vi "FipsAdjacent.vi"() -> (11 "Fips":i32[](array[numeric]))   [LabVIEW 2017] (continued)
 County, KY\"\t21075\t\"Hickman County, KY\"\t21105\n\"Fulton County, KY\"\t21075\t\"Mississippi County, MO\"\t29133\n\"Fulton County, KY\"\t21075\t\"New Madrid County, MO\"\t29143\n\"Fulton County, KY\"\t21075\t\"Lake County, TN\"\t47095\n\"Fulton County, KY\"\t21075\t\"Obion County, TN\"\t47131\n\"Gallatin County, KY\"\t21077\t\"Switzerland County, IN\"\t18155\n\"Gallatin County, KY\"\t21077\t\"Boone County, KY\"\t21015\n\"Gallatin County, KY\"\t21077\t\"Carroll County, KY\"\t21041\n\"Gallatin County, KY\"\t21077\t\"Gallatin County, KY\"\t21077\n\"Gallatin County, KY\"\t21077\t\"Grant County, KY\"\t21081\n\"Gallatin County, KY\"\t21077\t\"Owen County, KY\"\t21187\n\"Garrard County, KY\"\t21079\t\"Boyle County, KY\"\t21021\n\"Garrard County, KY\"\t21079\t\"Garrard County, KY\"\t21079\n\"Garrard County, KY\"\t21079\t\"Jessamine County, KY\"\t21113\n\"Garrard County, KY\"\t21079\t\"Lincoln County, KY\"\t21137\n\"Garrard County, KY\"\t21079\t\"Madison County, KY\"\t21151\n\"Garrard County, KY\"\t21079\t\"Mercer County, KY\"\t21167\n\"Garrard County, KY\"\t21079\t\"Rockcastle County, KY\"\t21203\n\"Grant County, KY\"\t21081\t\"Boone County, KY\"\t21015\n\"Grant County, KY\"\t21081\t\"Gallatin County, KY\"\t21077\n\"Grant County, KY\"\t21081\t\"Grant County, KY\"\t21081\n\"Grant County, KY\"\t21081\t\"Harrison County, KY\"\t21097\n\"Grant County, KY\"\t21081\t\"Kenton County, KY\"\t21117\n\"Grant County, KY\"\t21081\t\"Owen County, KY\"\t21187\n\"Grant County, KY\"\t21081\t\"Pendleton County, KY\"\t21191\n\"Grant County, KY\"\t21081\t\"Scott County, KY\"\t21209\n\"Graves County, KY\"\t21083\t\"Calloway County, KY\"\t21035\n\"Graves County, KY\"\t21083\t\"Carlisle County, KY\"\t21039\n\"Graves County, KY\"\t21083\t\"Graves County, KY\"\t21083\n\"Graves County, KY\"\t21083\t\"Hickman County, KY\"\t21105\n\"Graves County, KY\"\t21083\t\"McCracken County, KY\"\t21145\n\"Graves County, KY\"\t21083\t\"Marshall County, KY\"\t21157\n\"Graves County, KY\"\t21083\t\"Henry County, TN\"\t47079\n\"Graves County, KY\"\t21083\t\"Weakley County, TN\"\t47183\n\"Grayson County, KY\"\t21085\t\"Breckinridge County, KY\"\t21027\n\"Grayson County, KY\"\t21085\t\"Butler County, KY\"\t21031\n\"Grayson County, KY\"\t21085\t\"Edmonson County, KY\"\t21061\n\"Grayson County, KY\"\t21085\t\"Grayson County, KY\"\t21085\n\"Grayson County, KY\"\t21085\t\"Hardin County, KY\"\t21093\n\"Grayson County, KY\"\t21085\t\"Hart County, KY\"\t21099\n\"Grayson County, KY\"\t21085\t\"Ohio County, KY\"\t21183\n\"Green County, KY\"\t21087\t\"Adair County, KY\"\t21001\n\"Green County, KY\"\t21087\t\"Green County, KY\"\t21087\n\"Green County, KY\"\t21087\t\"Hart County, KY\"\t21099\n\"Green County, KY\"\t21087\t\"Larue County, KY\"\t21123\n\"Green County, KY\"\t21087\t\"Metcalfe County, KY\"\t21169\n\"Green County, KY\"\t21087\t\"Taylor County, KY\"\t21217\n\"Greenup County, KY\"\t21089\t\"Boyd County, KY\"\t21019\n\"Greenup County, KY\"\t21089\t\"Carter County, KY\"\t21043\n\"Greenup County, KY\"\t21089\t\"Greenup County, KY\"\t21089\n\"Greenup County, KY\"\t21089\t\"Lewis County, KY\"\t21135\n\"Greenup County, KY\"\t21089\t\"Lawrence County, OH\"\t39087\n\"Greenup County, KY\"\t21089\t\"Scioto County, OH\"\t39145\n\"Hancock County, KY\"\t21091\t\"Perry County, IN\"\t18123\n\"Hancock County, KY\"\t21091\t\"Spencer County, IN\"\t18147\n\"Hancock County, KY\"\t21091\t\"Breckinridge County, KY\"\t21027\n\"Hancock County, KY\"\t21091\t\"Daviess County, KY\"\t21059\n\"Hancock County, KY\"\t21091\t\"Hancock County, KY\"\t21091\n\"Hancock County, KY\"\t21091\t\"Ohio County, KY\"\t21183\n\"Hardin County, KY\"\t21093\t\"Harrison County, IN\"\t18061\n\"Hardin County, KY\"\t21093\t\"Breckinridge County, KY\"\t21027\n\"Hardin County, KY\"\t21093\t\"Bullitt County, KY\"\t21029\n\"Hardin County, KY\"\t21093\t\"Grayson County, KY\"\t21085\n\"Hardin County, KY\"\t21093\t\"Hardin County, KY\"\t21093\n\"Hardin County, KY\"\t21093\t\"Hart County, KY\"\t21099\n\"Hardin County, KY\"\t21093\t\"Jefferson County, KY\"\t21111\n\"Hardin County, KY\"\t21093\t\"Larue County, KY\"\t21123\n\"Hardin County, KY\"\t21093\t\"Meade County, KY\"\t21163\n\"Hardin County, KY\"\t21093\t\"Nelson County, KY\"\t21179\n\"Harlan County, KY\"\t21095\t\"Bell County, KY\"\t21013\n\"Harlan County, KY\"\t21095\t\"Harlan County, KY\"\t21095\n\"Harlan County, KY\"\t21095\t\"Leslie County, KY\"\t21131\n\"Harlan County, KY\"\t21095\t\"Letcher County, KY\"\t21133\n\"Harlan County, KY\"\t21095\t\"Perry County, KY\"\t21193\n\"Harlan County, KY\"\t21095\t\"Lee County, VA\"\t51105\n\"Harlan County, KY\"\t21095\t\"Wise County, VA\"\t51195\n\"Harrison County, KY\"\t21097\t\"Bourbon County, KY\"\t21017\n\"Harrison County, KY\"\t21097\t\"Bracken County, KY\"\t21023\n\"Harrison County, KY\"\t21097\t\"Grant County, KY\"\t21081\n\"Harrison County, KY\"\t21097\t\"Harrison County, KY\"\t21097\n\"Harrison County, KY\"\t21097\t\"Nicholas County, KY\"\t21181\n\"Harrison County, KY\"\t21097\t\"Pendleton County, KY\"\t21191\n\"Harrison County, KY\"\t21097\t\"Robertson County, KY\"\t21201\n\"Harrison County, KY\"\t21097\t\"Scott County, KY\"\t21209\n\"Hart County, KY\"\t21099\t\"Barren County, KY\"\t21009\n\"Hart County, KY\"\t21099\t\"Edmonson County, KY\"\t21061\n\"Hart County, KY\"\t21099\t\"Grayson County, KY\"\t21085\n\"Hart County, KY\"\t21099\t\"Green County, KY\"\t21087\n\"Hart County, KY\"\t21099\t\"Hardin County, KY\"\t21093\n\"Hart County, KY\"\t21099\t\"Hart County, KY\"\t21099\n\"Hart County, KY\"\t21099\t\"Larue County, KY\"\t21123\n\"Hart County, KY\"\t21099\t\"Metcalfe County, KY\"\t21169\n\"Henderson County, KY\"\t21101\t\"Posey County, IN\"\t18129\n\"Henderson County, KY\"\t21101\t\"Vanderburgh County, IN\"\t18163\n\"Henderson County, KY\"\t21101\t\"Warrick County, IN\"\t18173\n\"Henderson County, KY\"\t21101\t\"Daviess County, KY\"\t21059\n\"Henderson County, KY\"\t21101\t\"Henderson County, KY\"\t21101\n\"Henderson County, KY\"\t21101\t\"McLean County, KY\"\t21149\n\"Henderson County, KY\"\t21101\t\"Union County, KY\"\t21225\n\"Henderson County, KY\"\t21101\t\"Webster County, KY\"\t21233\n\"Henry County, KY\"\t21103\t\"Carroll County, KY\"\t21041\n\"Henry County, KY\"\t21103\t\"Franklin County, KY\"\t21073\n\"Henry County, KY\"\t21103\t\"Henry County, KY\"\t21103\n\"Henry County, KY\"\t21103\t\"Oldham County, KY\"\t21185\n\"Henry County, KY\"\t21103\t\"Owen County, KY\"\t21187\n\"Henry County, KY\"\t21103\t\"Shelby County, KY\"\t21211\n\"Henry County, KY\"\t21103\t\"Trimble County, KY\"\t21223\n\"Hickman County, KY\"\t21105\t\"Carlisle County, KY\"\t21039\n\"Hickman County, KY\"\t21105\t\"Fulton County, KY\"\t21075\n\"Hickman County, KY\"\t21105\t\"Graves County, KY\"\t21083\n\"Hickman County, KY\"\t21105\t\"Hickman County, KY\"\t21105\n\"Hickman County, KY\"\t21105\t\"Mississippi County, MO\"\t29133\n\"Hickman County, KY\"\t21105\t\"Obion County, TN\"\t47131\n\"Hickman County, KY\"\t21105\t\"Weakley County, TN\"\t47183\n\"Hopkins County, KY\"\t21107\t\"Caldwell County, KY\"\t21033\n\"Hopkins County, KY\"\t21107\t\"Christian County, KY\"\t21047\n\"Hopkins County, KY\"\t21107\t\"Hopkins County, KY\"\t21107\n\"Hopkins County, KY\"\t21107\t\"McLean County, KY\"\t21149\n\"Hopkins County, KY\"\t21107\t\"Muhlenberg County, KY\"\t21177\n\"Hopkins County, KY\"\t21107\t\"Webster County, KY\"\t21233\n\"Jackson County, KY\"\t21109\t\"Clay County, KY\"\t21051\n\"Jackson County, KY\"\t21109\t\"Estill County, KY\"\t21065\n\"Jackson County, KY\"\t21109\t\"Jackson County, KY\"\t21109\n\"Jackson County, KY\"\t21109\t\"Laurel County, KY\"\t21125\n\"Jackson County, KY\"\t21109\t\"Lee County, KY\"\t21129\n\"Jackson County, KY\"\t21109\t\"Madison County, KY\"\t21151\n\"Jackson County, KY\"\t21109\t\"Owsley County, KY\"\t21189\n\"Jackson County, KY\"\t21109\t\"Rockcastle County, KY\"\t21203\n\"Jefferson County, KY\"\t21111\t\"Clark County, IN\"\t18019\n\"Jefferson County, KY\"\t21111\t\"Floyd County, IN\"\t18043\n\"Jefferson County, KY\"\t21111\t\"Harrison County, IN\"\t18061\n\"Jefferson County, KY\"\t21111\t\"Bullitt County, KY\"\t21029\n\"Jefferson County, KY\"\t21111\t\"Hardin County, KY\"\t21093\n\"Jefferson County, KY\"\t21111\t\"Jefferson County, KY\"\t21111\n\"Jefferson County, KY\"\t21111\t\"Oldham County, KY\"\t21185\n\"Jefferson County, KY\"\t21111\t\"Shelby County, KY\"\t21211\n\"Jefferson County, KY\"\t21111\t\"Spencer County, KY\"\t21215\n\"Jessamine County, KY\"\t21113\t\"Fayette County, KY\"\t21067\n\"Jessamine County, KY\"\t21113\t\"Garrard County, KY\"\t21079\n\"Jessamine County, KY\"\t21113\t\"Jessamine County, KY\"\t21113\n\"Jessamine County, KY\"\t21113\t\"Madison County, KY\"\t21151\n\"Jessamine County, KY\"\t21113\t\"Mercer County, KY\"\t21167\n\"Jessamine County, KY\"\t21113\t\"Woodford County, KY\"\t21239\n\"Johnson County, KY\"\t21115\t\"Floyd County, KY\"\t21071\n\"Johnson County, KY\"\t21115\t\"Johnson County, KY\"\t21115\n\"Johnson County, KY\"\t21115\t\"Lawrence County, KY\"\t21127\n\"Johnson County, KY\"\t21115\t\"Magoffin County, KY\"\t21153\n\"Johnson County, KY\"\t21115\t\"Martin County, KY\"\t21159\n\"Johnson County, KY\"\t21115\t\"Morgan County, KY\"\t21175\n\"Kenton County, KY\"\t21117\t\"Boone County, KY\"\t21015\n\"Kenton County, KY\"\t21117\t\"Campbell County, KY\"\t21037\n\"Kenton County, KY\"\t21117\t\"Grant County, KY\"\t21081\n\"Kenton County, KY\"\t21117\t\"Kenton County, KY\"\t21117\n\"Kenton County, KY\"\t21117\t\"Pendleton County, KY\"\t21191\n\"Kenton County, KY\"\t21117\t\"Hamilton County, OH\"\t39061\n\"Knott County, KY\"\t21119\t\"Breathitt County, KY\"\t21025\n\"Knott County, KY\"\t21119\t\"Floyd County, KY\"\t21071\n\"Knott County, KY\"\t21119\t\"Knott County, KY\"\t21119\n\"Knott County, KY\"\t21119\t\"Letcher County, KY\"\t21133\n\"Knott County, KY\"\t21119\t\"Magoffin County, KY\"\t21153\n\"Knott County, KY\"\t21119\t\"Perry County, KY\"\t21193\n\"Knott County, KY\"\t21119\t\"Pike County, KY\"\t21195\n\"Knox County, KY\"\t21121\t\"Bell County, KY\"\t21013\n\"Knox County, KY\"\t21121\t\"Clay County, KY\"\t21051\n\"Knox County, KY\"\t21121\t\"Knox County, KY\"\t21121\n\"Knox County, KY\"\t21121\t\"Laurel County, KY\"\t21125\n\"Knox County, KY\"\t21121\t\"Whitley County, KY\"\t21235\n\"Larue County, KY\"\t21123\t\"Green County, KY\"\t21087\n\"Larue County, KY\"\t21123\t\"Hardin County, KY\"\t21093\n\"Larue County, KY\"\t21123\t\"Hart County, KY\"\t21099\n\"Larue County, KY\"\t21123\t\"Larue County, KY\"\t21123\n\"Larue County, KY\"\t21123\t\"Marion County, KY\"\t21155\n\"Larue County, KY\"\t21123\t\"Nelson County, KY\"\t21179\n\"Larue County, KY\"\t21123\t\"Taylor County, KY\"\t21217\n\"Laurel County, KY\"\t21125\t\"Clay County, KY\"\t21051\n\"Laurel County, KY\"\t21125\t\"Jackson County, KY\"\t21109\n\"Laurel County, KY\"\t21125\t\"Knox County, KY\"\t21121\n\"Laurel County, KY\"\t21125\t\"Laurel County, KY\"\t21125\n\"Laurel County, KY\"\t21125\t\"McCreary County, KY\"\t21147\n\"Laurel County, KY\"\t21125\t\"Pulaski County, KY\"\t21199\n\"Laurel County, KY\"\t21125\t\"Rockcastle County, KY\"\t21203\n\"Laurel County, KY\"\t21125\t\"Whitley County, KY\"\t21235\n\"Lawrence County, KY\"\t21127\t\"Boyd County, KY\"\t21019\n\"Lawrence County, KY\"\t21127\t\"Carter County, KY\"\t21043\n\"Lawrence County, KY\"\t21127\t\"Elliott County, KY\"\t21063\n\"Lawrence County, KY\"\t21127\t\"Johnson County, KY\"\t21115\n\"Lawrence County, KY\"\t21127\t\"Lawrence County, KY\"\t21127\n\"Lawrence County, KY\"\t21127\t\"Martin County, KY\"\t21159\n\"Lawrence County, KY\"\t21127\t\"Morgan County, KY\"\t21175\n\"Lawrence County, KY\"\t21127\t\"Wayne County, WV\"\t54099\n\"Lee County, KY\"\t21129\t\"Breathitt County, KY\"\t21025\n\"Lee County, KY\"\t21129\t\"Estill County, KY\"\t21065\n\"Lee County, KY\"\t21129\t\"Jackson County, KY\"\t21109\n\"Lee County, KY\"\t21129\t\"Lee County, KY\"\t21129\n\"Lee County, KY\"\t21129\t\"Owsley County, KY\"\t21189\n\"Lee County, KY\"\t21129\t\"Powell County, KY\"\t21197\n\"Lee County, KY\"\t21129\t\"Wolfe County, KY\"\t21237\n\"Leslie County, KY\"\t21131\t\"Bell County, KY\"\t21013\n\"Leslie County, KY\"\t21131\t\"Clay County, KY\"\t21051\n\"Leslie County, KY\"\t21131\t\"Harlan County, KY\"\t21095\n\"Leslie County, KY\"\t21131\t\"Leslie County, KY\"\t21131\n\"Leslie County, KY\"\t21131\t\"Perry County, KY\"\t21193\n\"Letcher County, KY\"\t21133\t\"Harlan County, KY\"\t21095\n\"Letcher County, KY\"\t21133\t\"Knott County, KY\"\t21119\n\"Letcher County, KY\"\t21133\t\"Letcher County, KY\"\t21133\n\"Letcher County, KY\"\t21133\t\"Perry County, KY\"\t21193\n\"Letcher County, KY\"\t21133\t\"Pike County, KY\"\t21195\n\"Letcher County, KY\"\t21133\t\"Wise County, VA\"\t51195\n\"Lewis County, KY\"\t21135\t\"Carter County, KY\"\t21043\n\"Lewis County, KY\"\t21135\t\"Fleming County, KY\"\t21069\n\"Lewis County, KY\"\t21135\t\"Greenup County, KY\"\t21089\n\"Lewis County, KY\"\t21135\t\"Lewis County, KY\"\t21135\n\"Lewis County, KY\"\t21135\t\"Mason County, KY\"\t21161\n\"Lewis County, KY\"\t21135\t\"Rowan County, KY\"\t21205\n\"Lewis County, KY\"\t21135\t\"Adams County, OH\"\t39001\n\"Lewis County, KY\"\t21135\t\"Scioto County, OH\"\t39145\n\"Lincoln County, KY\"\t21137\t\"Boyle County, KY\"\t21021\n\"Lincoln County, KY\"\t21137\t\"Casey County, KY\"\t21045\n\"Lincoln County, KY\"\t21137\t\"Garrard County, KY\"\t21079\n\"Lincoln County, KY\"\t21137\t\"Lincoln County, KY\"\t21137\n\"Lincoln County, KY\"\t21137\t\"Pulaski County, KY\"\t21199\n\"Lincoln County, KY\"\t21137\t\"Rockcastle County, KY\"\t21203\n\"Livingston County, KY\"\t21139\t\"Hardin County, IL\"\t17069\n\"Livingston County, KY\"\t21139\t\"Massac County, IL\"\t17127\n\"Livingston County, KY\"\t21139\t\"Pope County, IL\"\t17151\n\"Livingston County, KY\"\t21139\t\"Crittenden County, KY\"\t21055\n\"Livingston County, KY\"\t21139\t\"Livingston County, KY\"\t21139\n\"Livingston County, KY\"\t21139\t\"Lyon County, KY\"\t21143\n\"Livingston County, KY\"\t21139\t\"McCracken County, KY\"\t21145\n\"Livingston County, KY\"\t21139\t\"Marshall County, KY\"\t21157\n\"Logan County, KY\"\t21141\t\"Butler County, KY\"\t21031\n\"Logan County, KY\"\t21141\t\"Logan County, KY\"\t21141\n\"Logan County, KY\"\t21141\t\"Muhlenberg County, KY\"\t21177\n\"Logan County, KY\"\t21141\t\"Simpson County, KY\"\t21213\n\"Logan County, KY\"\t21141\t\"Todd County, KY\"\t21219\n\"Logan County, KY\"\t21141\t\"Warren County, KY\"\t21227\n\"Logan County, KY\"\t21141\t\"Robertson County, TN\"\t47147\n\"Lyon County, KY\"\t21143\t\"Caldwell County, KY\"\t21033\n\"Lyon County, KY\"\t21143\t\"Crittenden County, KY\"\t21055\n\"Lyon County, KY\"\t21143\t\"Livingston County, KY\"\t21139\n\"Lyon County, KY\"\t21143\t\"Lyon County, KY\"\t21143\n\"Lyon County, KY\"\t21143\t\"Marshall County, KY\"\t21157\n\"Lyon County, KY\"\t21143\t\"Trigg County, KY\"\t21221\n\"McCracken County, KY\"\t21145\t\"Massac County, IL\"\t17127\n\"McCracken County, KY\"\t21145\t\"Pulaski County, IL\"\t17153\n\"McCracken County, KY\"\t21145\t\"Ballard County, KY\"\t21007\n\"McCracken County, KY\"\t21145\t\"Carlisle County, KY\"\t21039\n\"McCracken County, KY\"\t21145\t\"Graves County, KY\"\t21083\n\"McCracken County, KY\"\t21145\t\"Livingston County, KY\"\t21139\n\"McCracken County, KY\"\t21145\t\"McCracken County, KY\"\t21145\n\"McCracken County, KY\"\t21145\t\"Marshall County, KY\"\t21157\n\"McCreary County, KY\"\t21147\t\"Laurel County, KY\"\t21125\n\"McCreary County, KY\"\t21147\t\"McCreary County, KY\"\t21147\n\"McCreary County, KY\"\t21147\t\"Pulaski County, KY\"\t21199\n\"McCreary County, KY\"\t21147\t\"Wayne County, KY\"\t21231\n\"McCreary County, KY\"\t21147\t\"Whitley County, KY\"\t21235\n\"McCreary County, KY\"\t21147\t\"Campbell County, TN\"\t47013\n\"McCreary County, KY\"\t21147\t\"Scott County, TN\"\t47151\n\"McLean County, KY\"\t21149\t\"Daviess County, KY\"\t21059\n\"McLean County, KY\"\t21149\t\"Henderson County, KY\"\t21101\n\"McLean County, KY\"\t21149\t\"Hopkins County, KY\"\t21107\n\"McLean County, KY\"\t21149\t\"McLean County, KY\"\t21149\n\"McLean County, KY\"\t21149\t\"Muhlenberg County, KY\"\t21177\n\"McLean County, KY\"\t21149\t\"Ohio County, KY\"\t21183\n\"McLean County, KY\"\t21149\t\"Webster County, KY\"\t21233\n\"Madison County, KY\"\t21151\t\"Clark County, KY\"\t21049\n\"Madison County, KY\"\t21151\t\"Estill County, KY\"\t21065\n\"Madison County, KY\"\t21151\t\"Fayette County, KY\"\t21067\n\"Madison County, KY\"\t21151\t\"Garrard County, KY\"\t21079\n\"Madison County, KY\"\t21151\t\"Jackson County, KY\"\t21109\n\"Madison County, KY\"\t21151\t\"Jessamine County, KY\"\t21113\n\"Madison County, KY\"\t21151\t\"Madison County, KY\"\t21151\n\"Madison County, KY\"\t21151\t\"Rockcastle County, KY\"\t21203\n\"Magoffin County, KY\"\t21153\t\"Breathitt County, KY\"\t21025\n\"Magoffin County, KY\"\t21153\t\"Floyd County, KY\"\t21071\n\"Magoffin County, KY\"\t21153\t\"Johnson County, KY\"\t21115\n\"Magoffin County, KY\"\t21153\t\"Knott County, KY\"\t21119\n\"Magoffin County, KY\"\t21153\t\"Magoffin County, KY\"\t21153\n\"Magoffin County, KY\"\t21153\t\"Morgan County, KY\"\t21175\n\"Magoffin County, KY\"\t21153\t\"Wolfe County, KY\"\t21237\n\"Marion County, KY\"\t21155\t\"Boyle County, KY\"\t21021\n\"Marion County, KY\"\t21155\t\"Casey County, KY\"\t21045\n\"Marion County, KY\"\t21155\t\"Larue County, KY\"\t21123\n\"Marion County, KY\"\t21155\t\"Marion County, KY\"\t21155\n\"Marion County, KY\"\t21155\t\"Nelson County, KY\"\t21179\n\"Marion County, KY\"\t21155\t\"Taylor County, KY\"\t21217\n\"Marion County, KY\"\t21155\t\"Washington County, KY\"\t21229\n\"Marshall County, KY\"\t21157\t\"Calloway County, KY\"\t21035\n\"Marshall County, KY\"\t21157\t\"Graves County, KY\"\t21083\n\"Marshall County, KY\"\t21157\t\"Livingston County, KY\"\t21139\n\"Marshall County, KY\"\t21157\t\"Lyon County, KY\"\t21143\n\"Marshall County, KY\"\t21157\t\"McCracken County, KY\"\t21145\n\"Marshall County, KY\"\t21157\t\"Marshall County, KY\"\t21157\n\"Marshall County, KY\"\t21157\t\"Trigg County, KY\"\t21221\n\"Martin County, KY\"\t21159\t\"Floyd County, KY\"\t21071\n\"Martin County, KY\"\t21159\t\"Johnson County, KY\"\t21115\n\"Martin County, KY\"\t21159\t\"Lawrence County, KY\"\t21127\n\"Martin County, KY\"\t21159\t\"Martin County, KY\"\t21159\n\"Martin County, KY\"\t21159\t\"Pike County, KY\"\t21195\n\"Martin County, KY\"\t21159\t\"Mingo County, WV\"\t54059\n\"Martin County, KY\"\t21159\t\"Wayne County, WV\"\t54099\n\"Mason County, KY\"\t21161\t\"Bracken County, KY\"\t21023\n\"Mason County, KY\"\t21161\t\"Fleming County, KY\"\t21069\n\"Mason County, KY\"\t21161\t\"Lewis County, KY\"\t21135\n\"Mason County, KY\"\t21161\t\"Mason County, KY\"\t21161\n\"Mason County, KY\"\t21161\t\"Robertson County, KY\"\t21201\n\"Mason County, KY\"\t21161\t\"Adams County, OH\"\t39001\n\"Mason County, KY\"\t21161\t\"Brown County, OH\"\t39015\n\"Meade County, KY\"\t21163\t\"Crawford County, IN\"\t18025\n\"Meade County, KY\"\t21163\t\"Harrison County, IN\"\t18061\n\"Meade County, KY\"\t21163\t\"Perry County, IN\"\t18123\n\"Meade County, KY\"\t21163\t\"Breckinridge County, KY\"\t21027\n\"Meade County, KY\"\t21163\t\"Hardin County, KY\"\t21093\n\"Meade County, KY\"\t21163\t\"Meade County, KY\"\t21163\n\"Menifee County, KY\"\t21165\t\"Bath County, KY\"\t21011\n\"Menifee County, KY\"\t21165\t\"Menifee County, KY\"\t21165\n\"Menifee County, KY\"\t21165\t\"Montgomery County, KY\"\t21173\n\"Menifee County, KY\"\t21165\t\"Morgan County, KY\"\t21175\n\"Menifee County, KY\"\t21165\t\"Powell County, KY\"\t21197\n\"Menifee County, KY\"\t21165\t\"Rowan County, KY\"\t21205\n\"Menifee County, KY\"\t21165\t\"Wolfe County, KY\"\t21237\n\"Mercer County, KY\"\t21167\t\"Anderson County, KY\"\t21005\n\"Mercer County, KY\"\t21167\t\"Boyle County, KY\"\t21021\n\"Mercer County, KY\"\t21167\t\"Garrard County, KY\"\t21079\n\"Mercer County, KY\"\t21167\t\"Jessamine County, KY\"\t21113\n\"Mercer County, KY\"\t21167\t\"Mercer County, KY\"\t21167\n\"Mercer County, KY\"\t21167\t\"Washington County, KY\"\t21229\n\"Mercer County, KY\"\t21167\t\"Woodford County, KY\"\t21239\n\"Metcalfe County, KY\"\t21169\t\"Adair County, KY\"\t21001\n\"Metcalfe County, KY\"\t21169\t\"Barren County, KY\"\t21009\n\"Metcalfe County, KY\"\t21169\t\"Cumberland County, KY\"\t21057\n\"Metcalfe County, KY\"\t21169\t\"Green County, KY\"\t21087\n\"Metcalfe County, KY\"\t21169\t\"Hart County, KY\"\t21099\n\"Metcalfe County, KY\"\t21169\t\"Metcalfe County, KY\"\t21169\n\"Metcalfe County, KY\"\t21169\t\"Monroe County, KY\"\t21171\n\"Monroe County, KY\"\t21171\t\"Allen County, KY\"\t21003\n\"Monroe County, KY\"\t21171\t\"Barren County, KY\"\t21009\n\"Monroe County, KY\"\t21171\t\"Cumberland County, KY\"\t21057\n\"Monroe County, KY\"\t21171\t\"Metcalfe County, KY\"\t21169\n\"Monroe County, KY\"\t21171\t\"Monroe County, KY\"\t21171\n\"Monroe County, KY\"\t21171\t\"Clay County, TN\"\t47027\n\"Monroe County, KY\"\t21171\t\"Macon County, TN\"\t47111\n\"Montgomery County, KY\"\t21173\t\"Bath County, KY\"\t21011\n\"Montgomery County, KY\"\t21173\t\"Bourbon County, KY\"\t21017\n\"Montgomery County, KY\"\t21173\t\"Clark County, KY\"\t21049\n\"Montgomery County, KY\"\t21173\t\"Menifee County, KY\"\t21165\n\"Montgomery County, KY\"\t21173\t\"Montgomery County, KY\"\t21173\n\"Montgomery County, KY\"\t21173\t\"Nicholas County, KY\"\t21181\n\"Montgomery County, KY\"\t21173\t\"Powell County, KY\"\t21197\n\"Morgan County, KY\"\t21175\t\"Elliott County, KY\"\t21063\n\"Morgan County, KY\"\t21175\t\"Johnson County, KY\"\t21115\n\"Morgan County, KY\"\t21175\t\"Lawrence County, KY\"\t21127\n\"Morgan County, KY\"\t21175\t\"Magoffin County, KY\"\t21153\n\"Morgan County, KY\"\t21175\t\"Menifee County, KY\"\t21165\n\"Morgan County, KY\"\t21175\t\"Morgan County, KY\"\t21175\n\"Morgan County, KY\"\t21175\t\"Rowan County, KY\"\t21205\n\"Morgan County, KY\"\t21175\t\"Wolfe County, KY\"\t21237\n\"Muhlenberg County, KY\"\t21177\t\"Butler County, KY\"\t21031\n\"Muhlenberg County, KY\"\t21177\t\"Christian County, KY\"\t21047\n\"Muhlenberg County, KY\"\t21177\t\"Hopkins County, KY\"\t21107\n\"Muhlenberg County, KY\"\t21177\t\"Logan County, KY\"\t21141\n\"Muhlenberg County, KY\"\t21177\t\"McLean County, KY\"\t21149\n\"Muhlenberg County, KY\"\t21177\t\"Muhlenberg County, KY\"\t21177\n\"Muhlenberg County, KY\"\t21177\t\"Ohio County, KY\"\t21183\n\"Muhlenberg County, KY\"\t21177\t\"Todd County, KY\"\t21219\n\"Nelson County, KY\"\t21179\t\"Anderson County, KY\"\t21005\n\"Nelson County, KY\"\t21179\t\"Bullitt County, KY\"\t21029\n\"Nelson County, KY\"\t21179\t\"Hardin County, KY\"\t21093\n\"Nelson County, KY\"\t21179\t\"Larue County, KY\"\t21123\n\"Nelson County, KY\"\t21179\t\"Marion County, KY\"\t21155\n\"Nelson County, KY\"\t21179\t\"Nelson County, KY\"\t21179\n\"Nelson County, KY\"\t21179\t\"Spencer County, KY\"\t21215\n\"Nelson County, KY\"\t21179\t\"Washington County, KY\"\t21229\n\"Nicholas County, KY\"\t21181\t\"Bath County, KY\"\t21011\n\"Nicholas County, KY\"\t21181\t\"Bourbon County, KY\"\t21017\n\"Nicholas County, KY\"\t21181\t\"Fleming County, KY\"\t21069\n\"Nicholas County, KY\"\t21181\t\"Harrison County, KY\"\t21097\n\"Nicholas County, KY\"\t21181\t\"Montgomery County, KY\"\t21173\n\"Nicholas County, KY\"\t21181\t\"Nicholas County, KY\"\t21181\n\"Nicholas County, KY\"\t21181\t\"Robertson County, KY\"\t21201\n\"Ohio County, KY\"\t21183\t\"Breckinridge County, KY\"\t21027\n\"Ohio County, KY\"\t21183\t\"Butler County, KY\"\t21031\n\"Ohio County, KY\"\t21183\t\"Daviess County, KY\"\t21059\n\"Ohio County, KY\"\t21183\t\"Grayson County, KY\"\t21085\n\"Ohio County, KY\"\t21183\t\"Hancock County, KY\"\t21091\n\"Ohio County, KY\"\t21183\t\"McLean County, KY\"\t21149\n\"Ohio County, KY\"\t21183\t\"Muhlenberg County, KY\"\t21177\n\"Ohio County, KY\"\t21183\t\"Ohio County, KY\"\t21183\n\"Oldham County, KY\"\t21185\t\"Clark County, IN\"\t18019\n\"Oldham County, KY\"\t21185\t\"Henry County, KY\"\t21103\n\"Oldham County, KY\"\t21185\t\"Jefferson County, KY\"\t21111\n\"Oldham County, KY\"\t21185\t\"Oldham County, KY\"\t21185\n\"Oldham County, KY\"\t21185\t\"Shelby County, KY\"\t21211\n\"Oldham County, KY\"\t21185\t\"Trimble County, KY\"\t21223\n\"Owen County, KY\"\t21187\t\"Carroll County, KY\"\t21041\n\"Owen County, KY\"\t21187\t\"Franklin County, KY\"\t21073\n\"Owen County, KY\"\t21187\t\"Gallatin County, KY\"\t21077\n\"Owen County, KY\"\t21187\t\"Grant County, KY\"\t21081\n\"Owen County, KY\"\t21187\t\"Henry County, KY\"\t21103\n\"Owen County, KY\"\t21187\t\"Owen County, KY\"\t21187\n\"Owen County, KY\"\t21187\t\"Scott County, KY\"\t21209\n\"Owsley County, KY\"\t21189\t\"Breathitt County, KY\"\t21025\n\"Owsley County, KY\"\t21189\t\"Clay County, KY\"\t21051\n\"Owsley County, KY\"\t21189\t\"Jackson County, KY\"\t21109\n\"Owsley County, KY\"\t21189\t\"Lee County, KY\"\t21129\n\"Owsley County, KY\"\t21189\t\"Owsley County, KY\"\t21189\n\"Owsley County, KY\"\t21189\t\"Perry County, KY\"\t21193\n\"Pendleton County, KY\"\t21191\t\"Bracken County, KY\"\t21023\n\"Pendleton County, KY\"\t21191\t\"Campbell County, KY\"\t21037\n\"Pendleton County, KY\"\t21191\t\"Grant County, KY\"\t21081\n\"Pendleton County, KY\"\t21191\t\"Harrison County, KY\"\t21097\n\"Pendleton County, KY\"\t21191\t\"Kenton County, KY\"\t21117\n\"Pendleton County, KY\"\t21191\t\"Pendleton County, KY\"\t21191\n\"Pendleton County, KY\"\t21191\t\"Clermont County, OH\"\t39025\n\"Perry County, KY\"\t21193\t\"Breathitt County, KY\"\t21025\n\"Perry County, KY\"\t21193\t\"Clay County, KY\"\t21051\n\"Perry County, KY\"\t21193\t\"Harlan County, KY\"\t21095\n\"Perry County, KY\"\t21193\t\"Knott County, KY\"\t21119\n\"Perry County, KY\"\t21193\t\"Leslie County, KY\"\t21131\n\"Perry County, KY\"\t21193\t\"Letcher County, KY\"\t21133\n\"Perry County, KY\"\t21193\t\"Owsley County, KY\"\t21189\n\"Perry County, KY\"\t21193\t\"Perry County, KY\"\t21193\n\"Pike County, KY\"\t21195\t\"Floyd County, KY\"\t21071\n\"Pike County, KY\"\t21195\t\"Knott County, KY\"\t21119\n\"Pike County, KY\"\t21195\t\"Letcher County, KY\"\t21133\n\"Pike County, KY\"\t21195\t\"Martin County, KY\"\t21159\n\"Pike County, KY\"\t21195\t\"Pike County, KY\"\t21195\n\"Pike County, KY\"\t21195\t\"Buchanan County, VA\"\t51027\n\"Pike County, KY\"\t21195\t\"Dickenson County, VA\"\t51051\n\"Pike County, KY\"\t21195\t\"Wise County, VA\"\t51195\n\"Pike County, KY\"\t21195\t\"Mingo County, WV\"\t54059\n\"Powell County, KY\"\t21197\t\"Clark County, KY\"\t21049\n\"Powell County, KY\"\t21197\t\"Estill County, KY\"\t21065\n\"Powell County, KY\"\t21197\t\"Lee County, KY\"\t21129\n\"Powell County, KY\"\t21197\t\"Menifee County, KY\"\t21165\n\"Powell County, KY\"\t21197\t\"Montgomery County, KY\"\t21173\n\"Powell County, KY\"\t21197\t\"Powell County, KY\"\t21197\n\"Powell County, KY\"\t21197\t\"Wolfe County, KY\"\t21237\n\"Pulaski County, KY\"\t21199\t\"Casey County, KY\"\t21045\n\"Pulaski County, KY\"\t21199\t\"Laurel County, KY\"\t21125\n\"Pulaski County, KY\"\t21199\t\"Lincoln County, KY\"\t21137\n\"Pulaski County, KY\"\t21199\t\"McCreary County, KY\"\t21147\n\"Pulaski County, KY\"\t21199\t\"Pulaski County, KY\"\t21199\n\"Pulaski County, KY\"\t21199\t\"Rockcastle County, KY\"\t21203\n\"Pulaski County, KY\"\t21199\t\"Russell County, KY\"\t21207\n\"Pulaski County, KY\"\t21199\t\"Wayne County, KY\"\t21231\n\"Robertson County, KY\"\t21201\t\"Bracken County, KY\"\t21023\n\"Robertson County, KY\"\t21201\t\"Fleming County, KY\"\t21069\n\"Robertson County, KY\"\t21201\t\"Harrison County, KY\"\t21097\n\"Robertson County, KY\"\t21201\t\"Mason County, KY\"\t21161\n\"Robertson County, KY\"\t21201\t\"Nicholas County, KY\"\t21181\n\"Robertson County, KY\"\t21201\t\"Robertson County, KY\"\t21201\n\"Rockcastle County, KY\"\t21203\t\"Garrard County, KY\"\t21079\n\"Rockcastle County, KY\"\t21203\t\"Jackson County, KY\"\t21109\n\"Rockcastle County, KY\"\t21203\t\"Laurel County, KY\"\t21125\n\"Rockcastle County, KY\"\t21203\t\"Lincoln County, KY\"\t21137\n\"Rockcastle County, KY\"\t21203\t\"Madison County, KY\"\t21151\n\"Rockcastle County, KY\"\t21203\t\"Pulaski County, KY\"\t21199\n\"Rockcastle County, KY\"\t21203\t\"Rockcastle County, KY\"\t21203\n\"Rowan County, KY\"\t21205\t\"Bath County, KY\"\t21011\n\"Rowan County, KY\"\t21205\t\"Carter County, KY\"\t21043\n\"Rowan County, KY\"\t21205\t\"Elliott County, KY\"\t21063\n\"Rowan County, KY\"\t21205\t\"Fleming County, KY\"\t21069\n\"Rowan County, KY\"\t21205\t\"Lewis County, KY\"\t21135\n\"Rowan County, KY\"\t21205\t\"Menifee County, KY\"\t21165\n\"Rowan County, KY\"\t21205\t\"Morgan County, KY\"\t21175\n\"Rowan County, KY\"\t21205\t\"Rowan County, KY\"\t21205\n\"Russell County, KY\"\t21207\t\"Adair County, KY\"\t21001\n\"Russell County, KY\"\t21207\t\"Casey County, KY\"\t21045\n\"Russell County, KY\"\t21207\t\"Clinton County, KY\"\t21053\n\"Russell County, KY\"\t21207\t\"Cumberland County, KY\"\t21057\n\"Russell County, KY\"\t21207\t\"Pulaski County, KY\"\t21199\n\"Russell County, KY\"\t21207\t\"Russell County, KY\"\t21207\n\"Russell County, KY\"\t21207\t\"Wayne County, KY\"\t21231\n\"Scott County, KY\"\t21209\t\"Bourbon County, KY\"\t21017\n\"Scott County, KY\"\t21209\t\"Fayette County, KY\"\t21067\n\"Scott County, KY\"\t21209\t\"Franklin County, KY\"\t21073\n\"Scott County, KY\"\t21209\t\"Grant County, KY\"\t21081\n\"Scott County, KY\"\t21209\t\"Harrison County, KY\"\t21097\n\"Scott County, KY\"\t21209\t\"Owen County, KY\"\t21187\n\"Scott County, KY\"\t21209\t\"Scott County, KY\"\t21209\n\"Scott County, KY\"\t21209\t\"Woodford County, KY\"\t21239\n\"Shelby County, KY\"\t21211\t\"Anderson County, KY\"\t21005\n\"Shelby County, KY\"\t21211\t\"Franklin County, KY\"\t21073\n\"Shelby County, KY\"\t21211\t\"Henry County, KY\"\t21103\n\"Shelby County, KY\"\t21211\t\"Jefferson County, KY\"\t21111\n\"Shelby County, KY\"\t21211\t\"Oldham County, KY\"\t21185\n\"Shelby County, KY\"\t21211\t\"Shelby County, KY\"\t21211\n\"Shelby County, KY\"\t21211\t\"Spencer County, KY\"\t21215\n\"Simpson County, KY\"\t21213\t\"Allen County, KY\"\t21003\n\"Simpson County, KY\"\t21213\t\"Logan County, KY\"\t21141\n\"Simpson County, KY\"\t21213\t\"Simpson County, KY\"\t21213\n\"Simpson County, KY\"\t21213\t\"Warren County, KY\"\t21227\n\"Simpson County, KY\"\t21213\t\"Robertson County, TN\"\t47147\n\"Simpson County, KY\"\t21213\t\"Sumner County, TN\"\t47165\n\"Spencer County, KY\"\t21215\t\"Anderson County, KY\"\t21005\n\"Spencer County, KY\"\t21215\t\"Bullitt County, KY\"\t21029\n\"Spencer County, KY\"\t21215\t\"Jefferson County, KY\"\t21111\n\"Spencer County, KY\"\t21215\t\"Nelson County, KY\"\t21179\n\"Spencer County, KY\"\t21215\t\"Shelby County, KY\"\t21211\n\"Spencer County, KY\"\t21215\t\"Spencer County, KY\"\t21215\n\"Taylor County, KY\"\t21217\t\"Adair County, KY\"\t21001\n\"Taylor County, KY\"\t21217\t\"Casey County, KY\"\t21045\n\"Taylor County, KY\"\t21217\t\"Green County, KY\"\t21087\n\"Taylor County, KY\"\t21217\t\"Larue County, KY\"\t21123\n\"Taylor County, KY\"\t21217\t\"Marion County, KY\"\t21155\n\"Taylor County, KY\"\t21217\t\"Taylor County, KY\"\t21217\n\"Todd County, KY\"\t21219\t\"Christian County, KY\"\t21047\n\"Todd County, KY\"\t21219\t\"Logan County, KY\"\t21141\n\"Todd County, KY\"\t21219\t\"Muhlenberg County, KY\"\t21177\n\"Todd County, KY\"\t21219\t\"Todd County, KY\"\t21219\n\"Todd County, KY\"\t21219\t\"Montgomery County, TN\"\t47125\n\"Todd County, KY\"\t21219\t\"Robertson County, TN\"\t47147\n\"Trigg County, KY\"\t21221\t\"Caldwell County, KY\"\t21033\n\"Trigg County, KY\"\t21221\t\"Calloway County, KY\"\t21035\n\"Trigg County, KY\"\t21221\t\"Christian County, KY\"\t21047\n\"Trigg County, KY\"\t21221\t\"Lyon County, KY\"\t21143\n\"Trigg County, KY\"\t21221\t\"Marshall County, KY\"\t21157\n\"Trigg County, KY\"\t21221\t\"Trigg County, KY\"\t21221\n\"Trigg County, KY\"\t21221\t\"Stewart County, TN\"\t47161\n\"Trimble County, KY\"\t21223\t\"Clark County, IN\"\t18019\n\"Trimble County, KY\"\t21223\t\"Jefferson County, IN\"\t18077\n\"Trimble County, KY\"\t21223\t\"Carroll County, KY\"\t21041\n\"Trimble County, KY\"\t21223\t\"Henry County, KY\"\t21103\n\"Trimble County, KY\"\t21223\t\"Oldham County, KY\"\t21185\n\"Trimble County, KY\"\t21223\t\"Trimble County, KY\"\t21223\n\"Union County, KY\"\t21225\t\"Gallatin County, IL\"\t17059\n\"Union County, KY\"\t21225\t\"Hardin County, IL\"\t17069\n\"Union County, KY\"\t21225\t\"Posey County, IN\"\t18129\n\"Union County, KY\"\t21225\t\"Crittenden County, KY\"\t21055\n\"Union County, KY\"\t21225\t\"Henderson County, KY\"\t21101\n\"Union County, KY\"\t21225\t\"Union County, KY\"\t21225\n\"Union County, KY\"\t21225\t\"Webster County, KY\"\t21233\n\"Warren County, KY\"\t21227\t\"Allen County, KY\"\t21003\n\"Warren County, KY\"\t21227\t\"Barren County, KY\"\t21009\n\"Warren County, KY\"\t21227\t\"Butler County, KY\"\t21031\n\"Warren County, KY\"\t21227\t\"Edmonson County, KY\"\t21061\n\"Warren County, KY\"\t21227\t\"Logan County, KY\"\t21141\n\"Warren County, KY\"\t21227\t\"Simpson County, KY\"\t21213\n\"Warren County, KY\"\t21227\t\"Warren County, KY\"\t21227\n\"Washington County, KY\"\t21229\t\"Anderson County, KY\"\t21005\n\"Washington County, KY\"\t21229\t\"Boyle County, KY\"\t21021\n\"Washington County, KY\"\t21229\t\"Marion County, KY\"\t21155\n\"Washington County, KY\"\t21229\t\"Mercer County, KY\"\t21167\n\"Washington County, KY\"\t21229\t\"Nelson County, KY\"\t21179\n\"Washington County, KY\"\t21229\t\"Washington County, KY\"\t21229\n\"Wayne County, KY\"\t21231\t\"Clinton County, KY\"\t21053\n\"Wayne County, KY\"\t21231\t\"McCreary County, KY\"\t21147\n\"Wayne County, KY\"\t21231\t\"Pulaski County, KY\"\t21199\n\"Wayne County, KY\"\t21231\t\"Russell County, KY\"\t21207\n\"Wayne County, KY\"\t21231\t\"Wayne County, KY\"\t21231\n\"Wayne County, KY\"\t21231\t\"Pickett County, TN\"\t47137\n\"Wayne County, KY\"\t21231\t\"Scott County, TN\"\t47151\n\"Webster County, KY\"\t21233\t\"Caldwell County, KY\"\t21033\n\"Webster County, KY\"\t21233\t\"Crittenden County, KY\"\t21055\n\"Webster County, KY\"\t21233\t\"Henderson County, KY\"\t21101\n\"Webster County, KY\"\t21233\t\"Hopkins County, KY\"\t21107\n\"Webster County, KY\"\t21233\t\"McLean County, KY\"\t21149\n\"Webster County, KY\"\t21233\t\"Union County, KY\"\t21225\n\"Webster County, KY\"\t21233\t\"Webster County, KY\"\t21233\n\"Whitley County, KY\"\t21235\t\"Bell County, KY\"\t21013\n\"Whitley County, KY\"\t21235\t\"Knox County, KY\"\t21121\n\"Whitley County, KY\"\t21235\t\"Laurel County, KY\"\t21125\n\"Whitley County, KY\"\t21235\t\"McCreary County, KY\"\t21147\n\"Whitley County, KY\"\t21235\t\"Whitley County, KY\"\t21235\n\"Whitley County, KY\"\t21235\t\"Campbell County, TN\"\t47013\n\"Whitley County, KY\"\t21235\t\"Claiborne County, TN\"\t47025\n\"Wolfe County, KY\"\t21237\t\"Breathitt County, KY\"\t21025\n\"Wolfe County, KY\"\t21237\t\"Lee County, KY\"\t21129\n\"Wolfe County, KY\"\t21237\t\"Magoffin County, KY\"\t21153\n\"Wolfe County, KY\"\t21237\t\"Menifee County, KY\"\t21165\n\"Wolfe County, KY\"\t21237\t\"Morgan County, KY\"\t21175\n\"Wolfe County, KY\"\t21237\t\"Powell County, KY\"\t21197\n\"Wolfe County, KY\"\t21237\t\"Wolfe County, KY\"\t21237\n\"Woodford County, KY\"\t21239\t\"Anderson County, KY\"\t21005\n\"Woodford County, KY\"\t21239\t\"Fayette County, KY\"\t21067\n\"Woodford County, KY\"\t21239\t\"Franklin County, KY\"\t21073\n\"Woodford County, KY\"\t21239\t\"Jessamine County, KY\"\t21113\n\"Woodford County, KY\"\t21239\t\"Mercer County, KY\"\t21167\n\"Woodford County, KY\"\t21239\t\"Scott County, KY\"\t21209\n\"Woodford County, KY\"\t21239\t\"Woodford County, KY\"\t21239\n\"Acadia Parish, LA\"\t22001\t\"Acadia Parish, LA\"\t22001\n\"Acadia Parish, LA\"\t22001\t\"Evangeline Parish, LA\"\t22039\n\"Acadia Parish, LA\"\t22001\t\"Jefferson Davis Parish, LA\"\t22053\n\"Acadia Parish, LA\"\t22001\t\"Lafayette Parish, LA\"\t22055\n\"Acadia Parish, LA\"\t22001\t\"St. Landry Parish, LA\"\t22097\n\"Acadia Parish, LA\"\t22001\t\"Vermilion Parish, LA\"\t22113\n\"Allen Parish, LA\"\t22003\t\"Allen Parish, LA\"\t22003\n\"Allen Parish, LA\"\t22003\t\"Beauregard Parish, LA\"\t22011\n\"Allen Parish, LA\"\t22003\t\"Evangeline Parish, LA\"\t22039\n\"Allen Parish, LA\"\t22003\t\"Jefferson Davis Parish, LA\"\t22053\n\"Allen Parish, LA\"\t22003\t\"Rapides Parish, LA\"\t22079\n\"Allen Parish, LA\"\t22003\t\"Vernon Parish, LA\"\t22115\n\"Ascension Parish, LA\"\t22005\t\"Ascension Parish, LA\"\t22005\n\"Ascension Parish, LA\"\t22005\t\"Assumption Parish, LA\"\t22007\n\"Ascension Parish, LA\"\t22005\t\"East Baton Rouge Parish, LA\"\t22033\n\"Ascension Parish, LA\"\t22005\t\"Iberville Parish, LA\"\t22047\n\"Ascension Parish, LA\"\t22005\t\"Livingston Parish, LA\"\t22063\n\"Ascension Parish, LA\"\t22005\t\"St. James Parish, LA\"\t22093\n\"Ascension Parish, LA\"\t22005\t\"St. John the Baptist Parish, LA\"\t22095\n\"Assumption Parish, LA\"\t22007\t\"Ascension Parish, LA\"\t22005\n\"Assumption Parish, LA\"\t22007\t\"Assumption Parish, LA\"\t22007\n\"Assumption Parish, LA\"\t22007\t\"Iberia Parish, LA\"\t22045\n\"Assumption Parish, LA\"\t22007\t\"Iberville Parish, LA\"\t22047\n\"Assumption Parish, LA\"\t22007\t\"Lafourche Parish, LA\"\t22057\n\"Assumption Parish, LA\"\t22007\t\"St. James Parish, LA\"\t22093\n\"Assumption Parish, LA\"\t22007\t\"St. Martin Parish, LA\"\t22099\n\"Assumption Parish, LA\"\t22007\t\"St. Mary Parish, LA\"\t22101\n\"Assumption Parish, LA\"\t22007\t\"Terrebonne Parish, LA\"\t22109\n\"Avoyelles Parish, LA\"\t22009\t\"Avoyelles Parish, LA\"\t22009\n\"Avoyelles Parish, LA\"\t22009\t\"Catahoula Parish, LA\"\t22025\n\"Avoyelles Parish, LA\"\t22009\t\"Concordia Parish, LA\"\t22029\n\"Avoyelles Parish, LA\"\t22009\t\"Evangeline Parish, LA\"\t22039\n\"Avoyelles Parish, LA\"\t22009\t\"La Salle Parish, LA\"\t22059\n\"Avoyelles Parish, LA\"\t22009\t\"Pointe Coupee Parish, LA\"\t22077\n\"Avoyelles Parish, LA\"\t22009\t\"Rapides Parish, LA\"\t22079\n\"Avoyelles Parish, LA\"\t22009\t\"St. Landry Parish, LA\"\t22097\n\"Avoyelles Parish, LA\"\t22009\t\"West Feliciana Parish, LA\"\t22125\n\"Beauregard Parish, LA\"\t22011\t\"Allen Parish, LA\"\t22003\n\"Beauregard Parish, LA\"\t22011\t\"Beauregard Parish, LA\"\t22011\n\"Beauregard Parish, LA\"\t22011\t\"Calcasieu Parish, LA\"\t22019\n\"Beauregard Parish, LA\"\t22011\t\"Jefferson Davis Parish, LA\"\t22053\n\"Beauregard Parish, LA\"\t22011\t\"Vernon Parish, LA\"\t22115\n\"Beauregard Parish, LA\"\t22011\t\"Newton County, TX\"\t48351\n\"Bienville Parish, LA\"\t22013\t\"Bienville Parish, LA\"\t22013\n\"Bienville Parish, LA\"\t22013\t\"Bossier Parish, LA\"\t22015\n\"Bienville Parish, LA\"\t22013\t\"Claiborne Parish, LA\"\t22027\n\"Bienville Parish, LA\"\t22013\t\"Jackson Parish, LA\"\t22049\n\"Bienville Parish, LA\"\t22013\t\"Lincoln Parish, LA\"\t22061\n\"Bienville Parish, LA\"\t22013\t\"Natchitoches Parish, LA\"\t22069\n\"Bienville Parish, LA\"\t22013\t\"Red River Parish, LA\"\t22081\n\"Bienville Parish, LA\"\t22013\t\"Webster Parish, LA\"\t22119\n\"Bienville Parish, LA\"\t22013\t\"Winn Parish, LA\"\t22127\n\"Bossier Parish, LA\"\t22015\t\"Lafayette County, AR\"\t05073\n\"Bossier Parish, LA\"\t22015\t\"Miller County, AR\"\t05091\n\"Bossier Parish, LA\"\t22015\t\"Bienville Parish, LA\"\t22013\n\"Bossier Parish, LA\"\t22015\t\"Bossier Parish, LA\"\t22015\n\"Bossier Parish, LA\"\t22015\t\"Caddo Parish, LA\"\t22017\n\"Bossier Parish, LA\"\t22015\t\"Red River Parish, LA\"\t22081\n\"Bossier Parish, LA\"\t22015\t\"Webster Parish, LA\"\t22119\n\"Caddo Parish, LA\"\t22017\t\"Miller County, AR\"\t05091\n\"Caddo Parish, LA\"\t22017\t\"Bossier Parish, LA\"\t22015\n\"Caddo Parish, LA\"\t22017\t\"Caddo Parish, LA\"\t22017\n\"Caddo Parish, LA\"\t22017\t\"De Soto Parish, LA\"\t22031\n\"Caddo Parish, LA\"\t22017\t\"Red River Parish, LA\"\t22081\n\"Caddo Parish, LA\"\t22017\t\"Cass County, TX\"\t48067\n\"Caddo Parish, LA\"\t22017\t\"Harrison County, TX\"\t48203\n\"Caddo Parish, LA\"\t22017\t\"Marion County, TX\"\t48315\n\"Caddo Parish, LA\"\t22017\t\"Panola County, TX\"\t48365\n\"Calcasieu Parish, LA\"\t22019\t\"Beauregard Parish, LA\"\t22011\n\"Calcasieu Parish, LA\"\t22019\t\"Calcasieu 
